vi "ShowData.vi"(11 "MessengerMCPU in":refnum<class "MessengerMCPU.lvclass">) -> (0 "abort":bool, 1 "acks":u32[](array[numeric]), 2 "subchannels":T2(array[cluster]), 3 "MessengerMCPU out":refnum<class "MessengerMCPU.lvclass">, 4 "lastID":u32)   [LabVIEW 2019, in "MessengerM.lvlib" / "MessengerMCPU.lvclass"]
uses:
  MessengerMCPU.lvclass
  Element.ctl
  MessengerM.lvlib
  SubChannelCPU/SubChannelCPU.lvclass
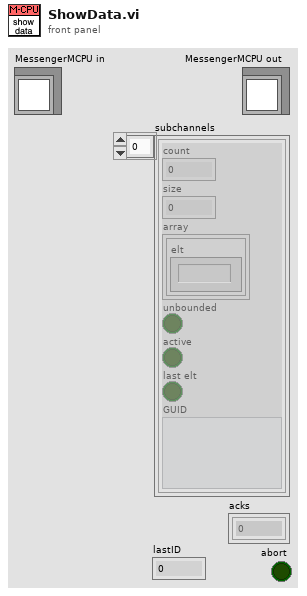
[diagram p1: front panel]
types:
  T1 = typedef "MessengerM.lvlib/Element.ctl" = string
  T2 = cluster{"count":i32, "size":i32, "array":cluster{"elt":T1}[], "unbounded":bool, "active":bool, "last elt":bool, "GUID":string}[]
  T3 = cluster{"GUID":string, "sub":refnum<class "SubChannelCPU.lvclass">}[]
  T4 = cluster{"count":i32, "size":i32, "array":cluster{"elt":T1}[], "unbounded":bool, "active":bool, "last elt":bool, "GUID":string}
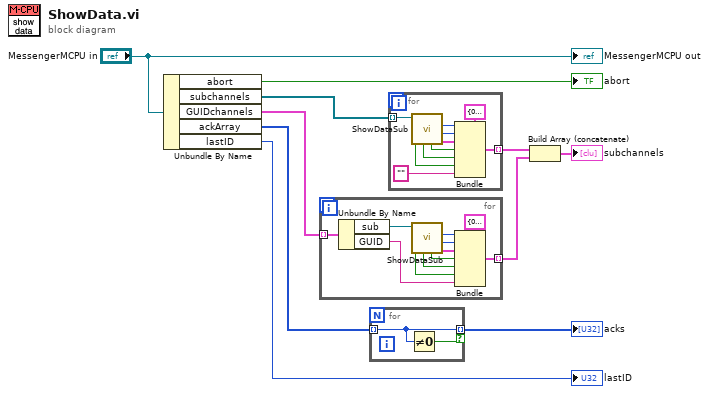
[diagram p0: block diagram]
diagram:
  n1 = Unbundle By Name("MessengerMCPU in") -> ("abort"=→"abort":bool, "subchannels"=w5:refnum<class "SubChannelCPU.lvclass">[], "GUIDchannels"=w3:T3, "ackArray"=w8:u32[], "lastID"=→"lastID":u32)
  n2 = for {
    tunnel: w3 -> [w21] mode=indexing
    tunnel: [w15] -> w1 mode=indexing
    n3 = Unbundle By Name(w21) -> ("sub"=w14:refnum<class "SubChannelCPU.lvclass">, "GUID"=w12:string)
    n4 = call-dynamic "ShowDataSub.vi"("SubChannel in"=w14) -> ("elements"=w18:cluster{"elt":T1}[], "size"=w19:i32, "count"=w20:i32, "unbounded"=w17:bool, "active"=w16:bool, "last element"=w11:bool)  [unwired: 4 in, 1 out]
    n5 = Bundle(cluster=T4 {"count"=0, "size"=0, "array"=[], "unbounded"=FALSE, "active"=FALSE, "last elt"=FALSE, "GUID"=""}, "count"=w20, "size"=w19, "array"=w18, "unbounded"=w17, "active"=w16, "last elt"=w11, "GUID"=w12) -> (w15:T4)
  }
  n6 = for {
    tunnel: w8 -> [w23] mode=indexing
    tunnel: [w23] -> w7 mode=indexing if=w22
    n7 = Not Equal To 0?(x=w23) -> (x != 0?=w22:bool)
  }
  "acks" <- w7
  n8 = for {
    tunnel: w5 -> [w33] mode=indexing
    tunnel: [w27] -> w4 mode=indexing
    n9 = call-dynamic "ShowDataSub.vi"("SubChannel in"=w33) -> ("elements"=w30:cluster{"elt":T1}[], "size"=w31:i32, "count"=w32:i32, "unbounded"=w29:bool, "active"=w28:bool, "last element"=w24:bool)  [unwired: 4 in, 1 out]
    n10 = Bundle(cluster=T4 {"count"=0, "size"=0, "array"=[], "unbounded"=FALSE, "active"=FALSE, "last elt"=FALSE, "GUID"=""}, "count"=w32, "size"=w31, "array"=w30, "unbounded"=w29, "active"=w28, "last elt"=w24, "GUID"="") -> (w27:T4)
  }
  n11 = Build Array (concatenate)(w4, w1) -> (→"subchannels":T2)
  "MessengerMCPU out" <- "MessengerMCPU in"
